vi "CRYGet Max Min from XY Graph Data.vi"(0 "Limits":u16(ring)=2 caption="茄拌" items=["Upper Only", "Lower Only", "Upper & Lower"], 1 "Limits Graph":refnum<vi>, 5 "Output failed":bool, 7 "X-Resolution":u8, 9 "Y-Resolution":u8, 11 "Tolerance":u16(ring)=2 caption="吝缴炼沥" items=["Individual Pts.", "Absolute Limits", "Floating Limits", "Floating Data", "Aligned Limits", "Aligned Data"], 12 "array of clusters":T1(array[cluster])) -> ()   [LabVIEW 2013]
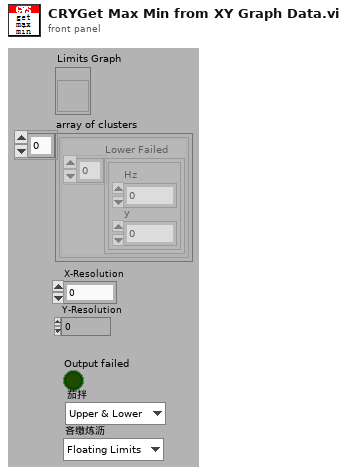
[diagram p1: front panel]
types:
  T1 = cluster{"Lower Failed":cluster{"Hz":dbl, "y":dbl}[]}[]
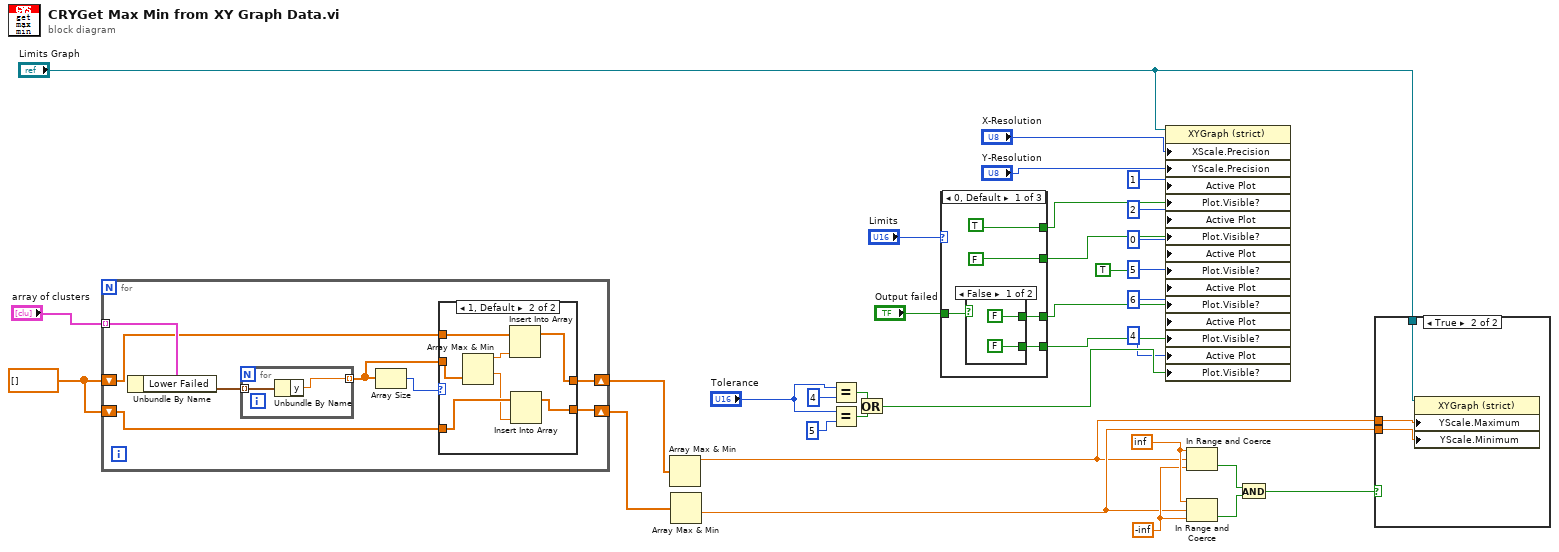
[diagram p0: block diagram]
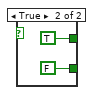
[diagram p3: hidden frame]
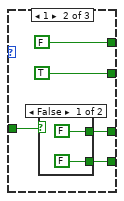
[diagram p4: hidden frame]
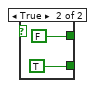
[diagram p5: hidden frame]
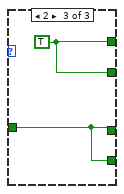
[diagram p6: hidden frame]
diagram:
  w7 = -inf
  w8 = inf
  w16 = dbl[] []
  n1 = for {
    tunnel: "array of clusters" -> [w41] mode=indexing
    shift-right: [w37] -> w33
    shift-left: w16 -> [w39]
    shift-right: [w35] -> w32
    shift-left: w16 -> [w38]
    n2 = Unbundle By Name(w41) -> ("Lower Failed"=w34:cluster{"Hz":dbl, "y":dbl}[])
    n3 = for {
      tunnel: w34 -> [w52] mode=indexing
      tunnel: [w51] -> w36 mode=indexing
      n4 = Unbundle By Name(w52) -> ("y"=w51:dbl)
    }
    n5 = Array Size(array=w36) -> (size(s)=w40:i32)
    n6 = case shown="1, Default" w40 {
      tunnel: w39 -> [w43 w50]
      tunnel: w38 -> [w42 w46]
      tunnel: [w43 w49] -> w37
      tunnel: [w42 w45] -> w35
      tunnel: w36 -> [_ w48]
      frame 0 {
      }
      frame 1, Default {
        n7 = Array Max & Min(array=w48) -> (max value=w47:dbl, min value=w44:dbl)  [unwired: 2 out]
        n8 = Insert Into Array(array=w50, new element=w47) -> (w49:dbl[])  [unwired: 1 in]
        n9 = Insert Into Array(array=w46, new element=w44) -> (w45:dbl[])  [unwired: 1 in]
      }
    }
  }
  n10 = Array Max & Min(array=w33) -> (max value=w2:dbl)  [unwired: 3 out]
  n11 = Array Max & Min(array=w32) -> (min value=w3:dbl)  [unwired: 3 out]
  n12 = Equal?(x="Tolerance", y=u16 4) -> (x = y?=w28:bool)
  n13 = Equal?(x="Tolerance", y=u16 5) -> (x = y?=w29:bool)
  n14 = Or(x=w28, y=w29) -> (x .or. y?=w24:bool)
  n15 = case shown="0, Default" "Limits" {
    tunnel: [TRUE ("Plot.Visible") FALSE ("Plot.Visible") w72] -> w23
    tunnel: [FALSE ("Plot.Visible") TRUE ("Plot.Visible") w72] -> w22
    tunnel: "Output failed" -> [w55 w64 w71]
    tunnel: [w54 w63 w71] -> w21
    tunnel: [w53 w62 w71] -> w20
    frame 0, Default {
      n16 = case shown="False" w55 {
        tunnel: [FALSE ("Plot.Visible") TRUE ("Plot.Visible")] -> w54
        tunnel: [FALSE ("Plot.Visible") FALSE ("Plot.Visible")] -> w53
        frame False {
        }
        frame True {
        }
      }
    }
    frame 1 {
      n17 = case shown="False" w64 {
        tunnel: [FALSE ("Plot.Visible") FALSE ("Plot.Visible")] -> w63
        tunnel: [FALSE ("Plot.Visible") TRUE ("Plot.Visible")] -> w62
        frame False {
        }
        frame True {
        }
      }
    }
    frame 2 {
      w72 = TRUE ("Plot.Visible")
    }
  }
  n18 = property on="Property Node" class="XYGraph (strict)"(reference="Limits Graph", "XScale.Precision"="X-Resolution", "YScale.Precision"="Y-Resolution", "Active Plot"=u32 1, "Plot.Visible?"=w23, "Active Plot"=u32 2, "Plot.Visible?"=w22, "Active Plot"=u32 0, "Plot.Visible?"=TRUE ("Plot.Visible"), "Active Plot"=u32 5, "Plot.Visible?"=w21, "Active Plot"=u32 6, "Plot.Visible?"=w20, "Active Plot"=u32 4, "Plot.Visible?"=w24) -> ()  [unwired: 1 in, 2 out]
  n19 = In Range and Coerce(upper limit=w8, x=w2, lower limit=w7) -> (In Range?=w6:bool)  [unwired: 1 out]
  n20 = In Range and Coerce(upper limit=w8, x=w3, lower limit=w7) -> (In Range?=w5:bool)  [unwired: 1 out]
  n21 = And(x=w6, y=w5) -> (x .and. y?=w4:bool)
  n22 = case shown="True" w4 {
    tunnel: w3 -> [_ w75]
    tunnel: w2 -> [_ w74]
    tunnel: "Limits Graph" -> [_ w73]
    frame False {
    }
    frame True {
      n23 = property on="Property Node" class="XYGraph (strict)"(reference=w73, "YScale.Maximum"=w74, "YScale.Minimum"=w75) -> ()  [unwired: 1 in, 2 out]
    }
  }
